vi "2.vi"() -> ()   [LabVIEW 2020]
uses:
  <vilib>/Utility/file.llb/Read Delimited Spreadsheet (DBL).vi
  <vilib>/Utility/file.llb/Write Delimited Spreadsheet (DBL).vi
panel:
  out "White LED spectrum":cluster{"Y":dbl[], "Y":dbl[]}[](graph)
  in  "file path of modified data":path
  out "modified data":dbl[][](array[numeric])
  out "Average count below 400nm":dbl
  out "original data":dbl[][](array[numeric])
  in  "file path of original data":path
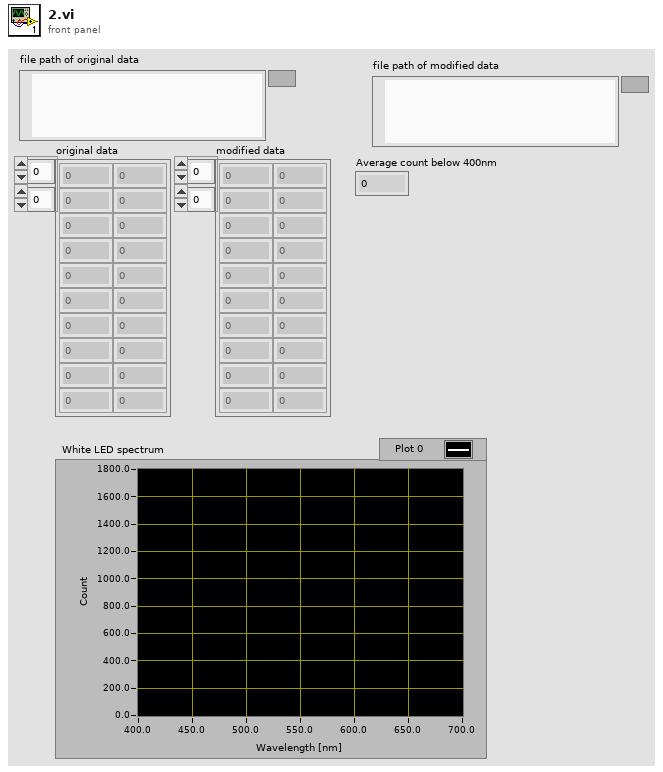
[diagram p1: front panel]
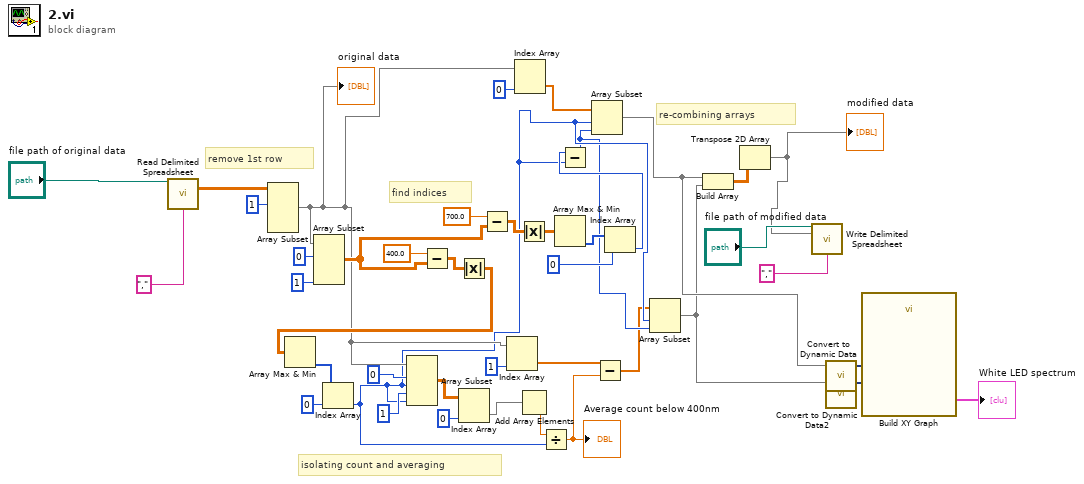
[diagram p0: block diagram]
diagram:
  # "isolating count and averaging"
  # "re-combining arrays"
  # "find indices"
  # "remove 1st row"
  n1 = call-poly <vilib>:"Read Delimited Spreadsheet.vi"("file path (dialog if empty)"="file path of original data", "delimiter (\\t)"="," ("delimiter (\\t)")) -> ("all rows"=w40:dbl[][])  [unwired: 8 in, 5 out]
  n2 = Array Subset(array=w40, index (row)=1 ("index")) -> (w15:dbl[][])  [unwired: 3 in]
  "original data" <- w15
  n3 = Array Subset(array=w15, index (row)=0 ("index"), length (col)=1 ("length")) -> (w20:dbl[][])  [unwired: 2 in]
  n4 = Subtract(x=400.0, y=w20) -> (x-y=w35:dbl[][])
  n5 = Absolute Value(x=w35) -> (abs(x)=w34:dbl[][])
  n6 = Array Max & Min(array=w34) -> (min index (indices)=w33:i32[])  [unwired: 3 out]
  n7 = Index Array(array=w33, index=0) -> (element=w8:i32)
  n8 = Array Subset(array=w15, index (row)=0 ("index"), length (row)=w8, index (col)=1 ("index"), length (col)=w8) -> (w29:dbl[][])
  n9 = Index Array(array=w29, index (col)=0 ("disabled index (col)")) -> (element=w27:dbl[])  [unwired: 1 in]
  n10 = Subtract(x=700.0, y=w20) -> (x-y=w21:dbl[][])
  n11 = Index Array(array=w15, index (col)=1 ("disabled index (col)")) -> (element=w24:dbl[])  [unwired: 1 in]
  n12 = Index Array(array=w15, index (col)=0) -> (element=w14:dbl[])  [unwired: 1 in]
  n13 = Absolute Value(x=w21) -> (abs(x)=w19:dbl[][])
  n14 = Add Array Elements(numeric array=w27) -> (sum=w26:dbl)
  n15 = Divide(x=w26, y=w8) -> (x/y=w23:dbl)
  "Average count below 400nm" <- w23
  n16 = Array Max & Min(array=w19) -> (min index (indices)=w18:i32[])  [unwired: 3 out]
  n17 = Subtract(x=w24, y=w23) -> (x-y=w6:dbl[])
  n18 = Index Array(array=w18, index=0) -> (element=w13:i32)
  n19 = Subtract(x=w13, y=w8) -> (x-y=w7:i32)
  n20 = Array Subset(array=w14, index=w8, length=w7) -> (w4:dbl[])
  n21 = Array Subset(array=w6, index=w8, length=w7) -> (w2:dbl[])
  n22 = Build Array(w4, w2) -> (w10:dbl[][])
  n23 = Transpose 2D Array(2D array=w10) -> (transposed array=w9:dbl[][])
  "modified data" <- w9
  n24 = call-poly <vilib>:"Write Delimited Spreadsheet.vi"("file path (dialog if empty)"="file path of modified data", "2D data"=w9, "delimiter (\\t)"="," ("delimiter (\\t)")) -> ()  [unwired: 11 in, 2 out]
  n25 = call "Convert to Dynamic Data"("Array"=w4) -> ("Dynamic Data Type"=w3:dynamicdata)  [unwired: 3 in]
  n26 = call "Convert to Dynamic Data2"("Array"=w2) -> ("Dynamic Data Type"=w1:dynamicdata)  [unwired: 3 in]
  n27 = call "Build XY Graph"("Y Input"=w1, "X Input"=w3) -> ("XY Graph"=→"White LED spectrum":cluster{"X":dbl[], "Y":dbl[]}[])  [unwired: 8 in, 1 out]
